vi "ns-to-tick-converter.vi"(10 "Gated-2  (ns)2":i64, 11 "Delay-2 (ns)":i64) -> (2 "Numeric":i64, 3 "Numeric 2":i64)   [LabVIEW 2018]
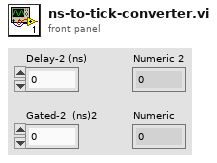
[diagram p1: front panel]
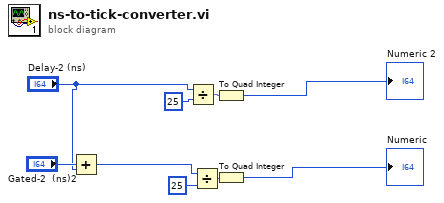
[diagram p0: block diagram]
diagram:
  n1 = Add(x="Gated-2  (ns)2", y="Delay-2 (ns)") -> (x+y=w2:i64)
  n2 = Divide(x="Delay-2 (ns)", y=i64 25) -> (x/y=w3:fxp<+,32,16>)
  n3 = Divide(x=w2, y=i64 25) -> (x/y=w6:fxp<+,32,16>)
  n4 = To Quad Integer(1:w3) -> (0:→"Numeric 2":i64)
  n5 = To Quad Integer(1:w6) -> (0:→"Numeric":i64)
